vi "Initialize.vi"(9 "State Variables in":T1, 10 "Item.Data":T8, 11 "NIVS.Gateway IP Address":string) -> (0 "error out":errorcluster, 3 "State Variables out":T1)   [LabVIEW 2020, in "Instrument Workspace Shared.lvlib"]
uses:
  Instrument Workspace Shared.lvlib
  Types/State Variables.ctl
  <vilib>/NI VeriStand/Execution/Workspace/WorkspaceAPI.ctl
  NationalInstruments.VeriStand.ClientAPI
  NationalInstruments.VeriStand.SystemStorage
  <vilib>/NI VeriStand/Display Template Support/DisplayTemplateSupport.llb/enum_Display Template Handler Minimal To Workspace.ctl
  <vilib>/NI VeriStand/Display Template Support/DisplayTemplateSupport.llb/enum_Display Template Handler Minimal To Widget Msg.ctl
  <vilib>/NI/STM/TCP/TCP Connection Info.ctl
  <vilib>/NI/STM/SubVIs/MetaDataElement.ctl
  Types/CD Saved State.ctl
  <vilib>/NI VeriStand/Execution/Workspace/SystemStateEventRef.ctl
  <vilib>/NI VeriStand/Execution/Workspace/Target State Info.ctl
  <vilib>/NI VeriStand/Execution/Workspace/Target State.ctl
  <vilib>/NI VeriStand/Execution/Workspace/SystemStateRegEventRef.ctl
  <vilib>/NI VeriStand/Display Template Support/DisplayTemplateSupport.llb/cluster_Screen Item Settings.ctl
  <vilib>/NI VeriStand/Display Template Support/DisplayTemplateSupport.llb/cluster_Graph Scale Settings.ctl
  <vilib>/NI VeriStand/Display Template Support/DisplayTemplateSupport.llb/cluster_Graph Plot Settings.ctl
  <vilib>/NI VeriStand/Execution/Workspace/NI_VS Workspace ExecutionAPI.lvlib
  <vilib>/NI/STM/NI STM.lvlib
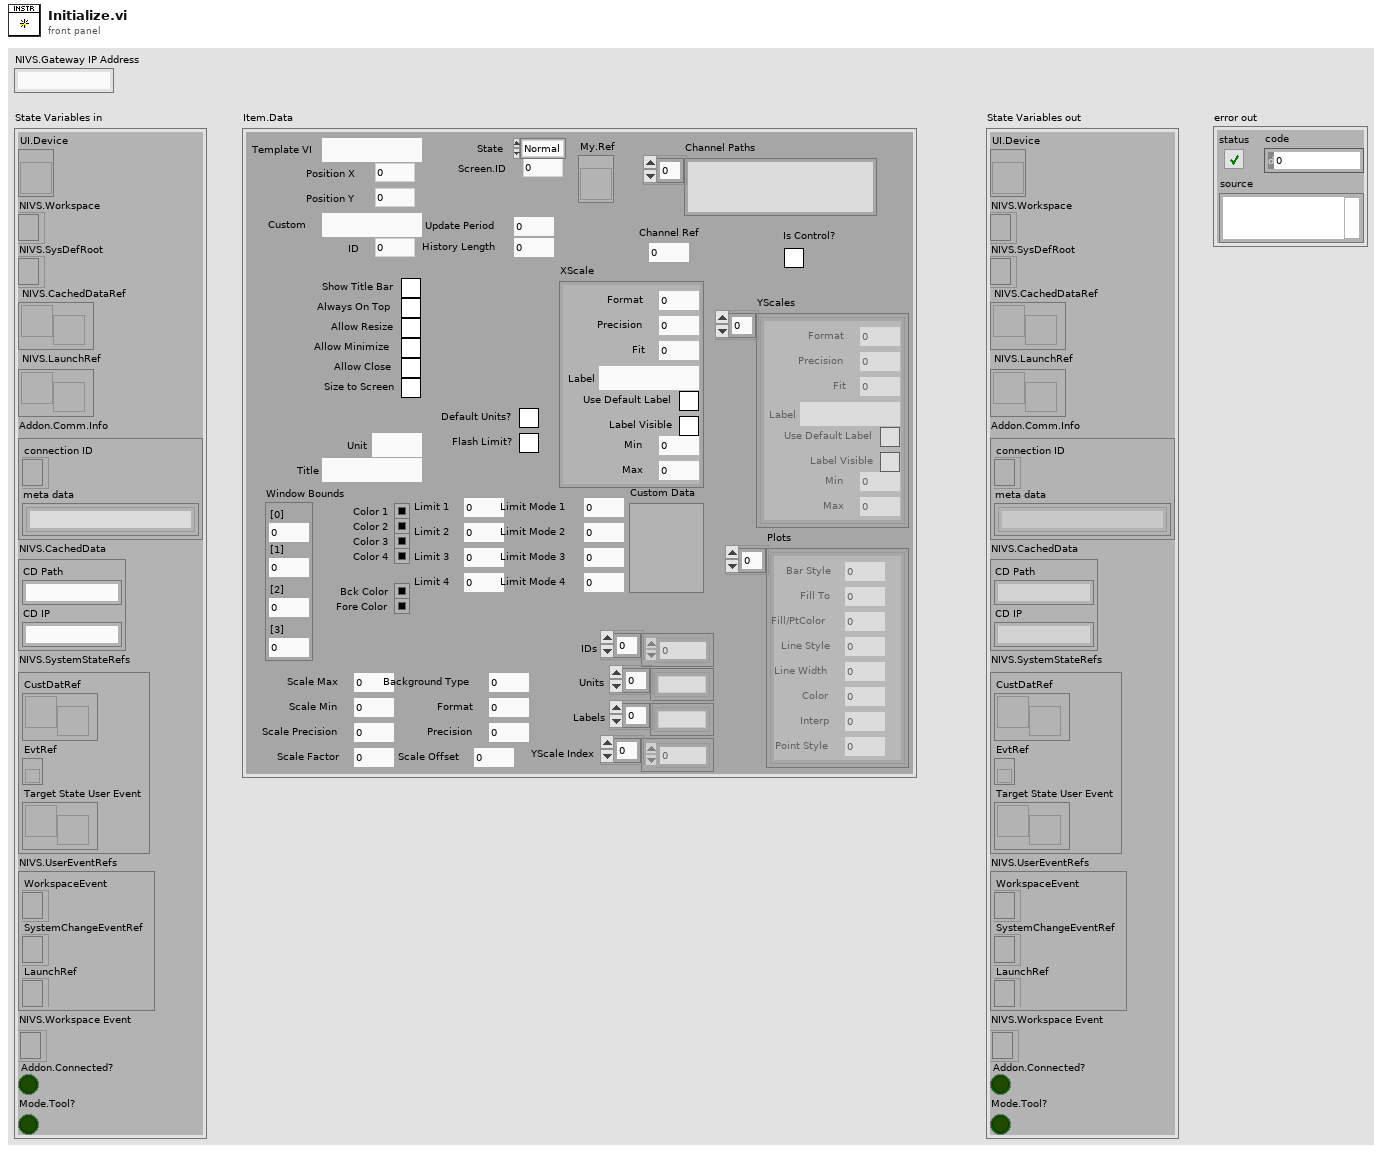
[diagram p1: front panel]
types:
  T1 = typedef "Instrument Workspace Shared.lvlib/State Variables.ctl" = cluster{"UI.Device":refnum<vi>, "NIVS.Workspace":T2, "NIVS.SysDefRoot":refnum<k24>, "NIVS.CachedDataRef":refnum<user-event>, "NIVS.LaunchRef":refnum<user-event>, "Addon.Comm.Info":T3, "NIVS.CachedData":T5, "NIVS.SystemStateRefs":T6, "NIVS.UserEventRefs":cluster{"WorkspaceEvent":refnum<event-registration>, "SystemChangeEventRef":T7, "LaunchRef":refnum<event-registration>}, "NIVS.Workspace Event":refnum<event-registration>, "Addon.Connected?":bool, "Mode.Tool?":bool}
  T2 = typedef "NI_VS Workspace ExecutionAPI.lvlib/WorkspaceAPI.ctl" = refnum<k24>
  T3 = typedef "NI STM.lvlib/TCP Connection Info.ctl" = cluster{"connection ID":refnum<k5>, "meta data":T4[]}
  T4 = typedef "NI STM.lvlib/MetaDataElement.ctl" = string
  T5 = typedef "Instrument Workspace Shared.lvlib/CD Saved State.ctl" = cluster{"CD Path":string, "CD IP":string}
  T6 = typedef "NI_VS Workspace ExecutionAPI.lvlib/SystemStateEventRef.ctl" = cluster{"CustDatRef":refnum<user-event>, "EvtRef":refnum<k27>, "Target State User Event":refnum<user-event>}
  T7 = typedef "NI_VS Workspace ExecutionAPI.lvlib/SystemStateRegEventRef.ctl" = refnum<event-registration>
  T8 = typedef "cluster_Screen Item Settings.ctl" = cluster{"Template VI":string, "Position X":i32, "Position Y":i32, "Custom":string, "Show Title Bar":bool, "ID":i32, "Always On Top":bool, "Allow Resize":bool, "Allow Minimize":bool, "Allow Close":bool, "Size to Screen":bool, "Screen.ID":i32, "State":enum16{"Normal", "New"}, "Title":string, "Window Bounds":cluster{"[0]":i16, "[1]":i16, "[2]":i16, "[3]":i16}, "Channel Ref":u64, "Unit":string, "Default Units?":bool, "Flash Limit?":bool, "Color 1":u32, "Color 2":u32, "Color 3":u32, "Color 4":u32, "Bck Color":u32, "Fore Color":u32, "Limit 1":dbl, "Limit 2":dbl, "Limit 3":dbl, "Limit 4":dbl, "Limit Mode 1":i32, "Limit Mode 2":i32, "Limit Mode 3":i32, "Limit Mode 4":i32, "Scale Precision":i32, "Scale Min":dbl, "Scale Max":dbl, "Format":i32, "Precision":i32, "Background Type":i32, "IDs":i32[], "Units":string[], "Labels":string[], "Scale Factor":dbl, "Scale Offset":dbl, "YScale Index":u32[], "XScale":T9, "YScales":T9[], "Plots":T10[], "Update Period":dbl, "History Length":dbl, "My.Ref":refnum<vi>, "Is Control?":bool, "Channel Paths":string[], "Custom Data":variant}
  T9 = typedef "cluster_Graph Scale Settings.ctl" = cluster{"Format":u8, "Precision":u8, "Fit":u8, "Label":string, "Use Default Label":bool, "Label Visible":bool, "Min":dbl, "Max":dbl}
  T10 = typedef "cluster_Graph Plot Settings.ctl" = cluster{"Bar Style":u8, "Fill To":i16, "Fill/PtColor":u32, "Line Style":u8, "Line Width":u8, "Color":u32, "Interp":u8, "Point Style":u8}
  T11 = cluster{"NIVS.Workspace Event":refnum<event-registration>, "SystemChangeEventRef":T7, "Event Registration Refnum":refnum<event-registration>}
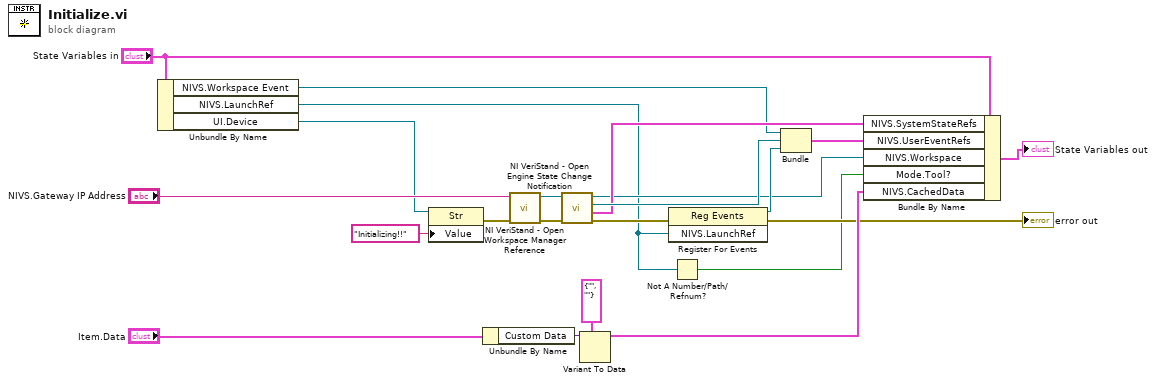
[diagram p0: block diagram]
diagram:
  n1 = Unbundle By Name("State Variables in") -> ("NIVS.Workspace Event"=w8:refnum<event-registration>, "NIVS.LaunchRef"=w2:refnum<user-event>, "UI.Device"=w5:refnum<vi>)
  n2 = property class="Str"(reference=w5, "Value"="Initializing!!") -> (error out=w4:errorcluster)  [unwired: 1 in, 1 out]
  n3 = Unbundle By Name("Item.Data") -> ("Custom Data"=w18:variant)
  n4 = call <vilib>:"NI VeriStand - Open Workspace Manager Reference.vi"("error in (no error)"=w4, "Gateway IP Address (\"\": localhost)"="NIVS.Gateway IP Address") -> ("error out"=w20:errorcluster, "WorkspaceManager"=w21:T2)  [unwired: 8 in]
  n5 = call <vilib>:"NI VeriStand - Open Engine State Change Notification.vi"("error in (no error)"=w20, "WorkspaceManager in"=w21) -> ("error out"=w17:errorcluster, "SystemStateRefs"=w12:T6, "SystemChangeEventRef"=w14:T7, "WorkspaceManager out"=w6:T2)  [unwired: 6 in]
  n6 = Variant To Data(type=T5 {"CD Path"="", "CD IP"=""}, Variant=w18) -> (data=w9:T5)  [unwired: 1 in, 1 out]
  n7 = register-events(error in=w17, w2) -> (reference out=w22:refnum<event-registration>, error out=→"error out":errorcluster)  [unwired: 1 in]
  n8 = Not A Number/Path/Refnum?(number/path/refnum=w2) -> (NaN/Path/Refnum?=w1:bool)
  n9 = Bundle("NIVS.Workspace Event"=w8, "SystemChangeEventRef"=w14, "Event Registration Refnum"=w22) -> (w11:T11)  [unwired: 1 in]
  n10 = Bundle By Name(cluster="State Variables in", "NIVS.SystemStateRefs"=w12, "NIVS.UserEventRefs"=w11, "NIVS.Workspace"=w6, "Mode.Tool?"=w1, "NIVS.CachedData"=w9) -> (→"State Variables out":T1)
